vi "Test Quaternion SLERP.vi"(11 "Test Case In":refnum<class "AR.lvclass">) -> (0 "error out":errorcluster, 3 "Test Case Out":refnum<class "AR.lvclass">)   [LabVIEW 2020, in "g_ar_toolkit.test.lvlib" / "AR.lvclass"]
uses:
  AR.lvclass
  C:/Program Files (x86)/National Instruments/LabVIEW 2020/vi.lib/Astemes/LUnit/Test Case.lvclass
  g_ar_toolkit.ar/Quaternion.ctl
  <vilib>/Astemes/LUnit/Test Case.lvclass/Test Case.ctl
  <vilib>/Astemes/LUnit/Append Fail Result.vi
  <vilib>/Astemes/LUnit/Append Pass Result.vi
  <vilib>/Astemes/LUnit/Run In UI.vi
  <vilib>/Utility/error.llb/Clear Errors.vi
  g_ar_toolkit.common/Module Path.vi
  <vilib>/Utility/error.llb/Error Cluster From Error Code.vi
  AR.lvclass/AR.ctl
  g_ar_toolkit.ar/g_ar_toolkit.ar.lvlib
  <vilib>/Astemes/LUnit/Test Case.lvclass
  C:/Program Files (x86)/National Instruments/LabVIEW 2020/vi.lib/Astemes/LUnit/LUnit Runnable.lvclass
  C:/serenial/libraries/g-augmented-reality-toolkit/LabVIEW/g_ar_toolkit.test/ar/AR.lvclass
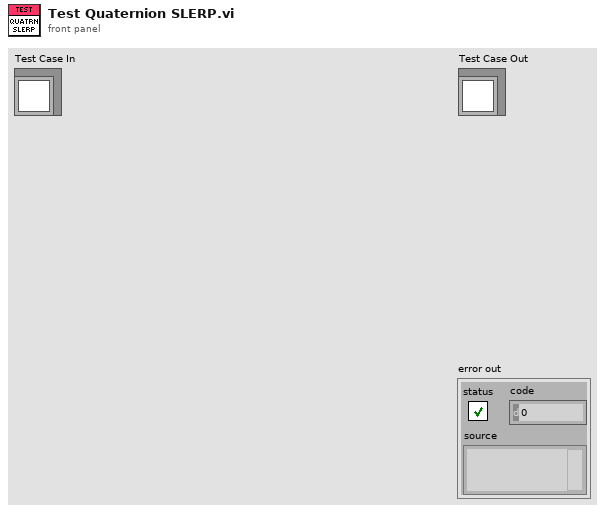
[diagram p1: front panel]
types:
  T1 = typedef "g_ar_toolkit.ar.lvlib/Quaternion.ctl" = cluster{"w":dbl, "x":dbl, "y":dbl, "z":dbl}
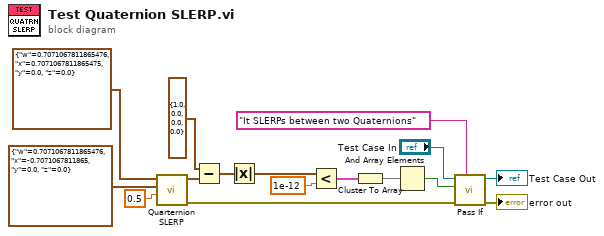
[diagram p0: block diagram]
diagram:
  n1 = call "Quarternion SLERP.vi"("Factor"=0.5, "To"=T1 {"w"=0.7071067811865476, "x"=-0.7071067811865, "y"=0.0, "z"=0.0} ("Quaternion"), "From"=T1 {"w"=0.7071067811865476, "x"=0.7071067811865475, "y"=0.0, "z"=0.0} ("Quaternion")) -> ("error out"=w13:errorcluster, "SLERP Result"=w4:T1)  [unwired: 7 in]
  n2 = Subtract ("Subtract.vi")(x=T1 {"w"=1.0, "x"=0.0, "y"=0.0, "z"=0.0} ("Quaternion"), y=w4) -> (x-y=w9:T1)
  n3 = Absolute Value ("Absolute Value.vi")(x=w9) -> (abs(x)=w8:T1)
  n4 = Less?(x=w8, y=1e-12) -> (x < y?=w6:cluster{"w":bool, "x":bool, "y":bool, "z":bool})
  n5 = Cluster To Array(cluster=w6) -> (array=w3:bool[])
  n6 = And Array Elements(Boolean array=w3) -> (logical AND=w2:bool)
  n7 = call <vilib>:"Pass If.vi"("Description"="It SLERPs between two Quaternions", "error in (no error)"=w13, "Pass?"=w2, "LUnit Test Case In"="Test Case In") -> ("error out"=→"error out":errorcluster, "LUnit Test Case Out"=→"Test Case Out":refnum<class "AR.lvclass">)  [unwired: 6 in]
